vi "MotorTypeParametersMaxMin.vi"(11 "MotorType":T2) -> (2 "Min":T1, 3 "Max":T1)   [LabVIEW 2019, in "CubeMarsBLDClib.lvlib"]
uses:
  CubeMarsBLDClib.lvlib
  MotorType.ctl
  MotorParameters.ctl
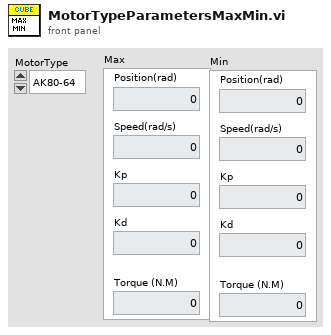
[diagram p1: front panel]
types:
  T1 = typedef "CubeMarsBLDClib.lvlib/MotorParameters.ctl" = cluster{"Position(rad)":dbl, "Speed(rad/s)":dbl, "Kp":dbl, "Kd":dbl, "Torque (N.M)":dbl}
  T2 = typedef "CubeMarsBLDClib.lvlib/MotorType.ctl" = enum16{"AK80-64", "AK80-9", "AK80-8", "AK80-6", "AK70-10", "AK60-6", "AK10-9"}
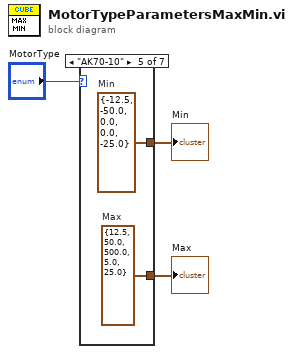
[diagram p0: block diagram]
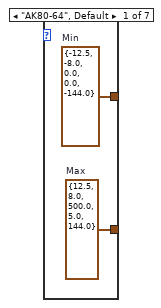
[diagram p2: hidden frame]
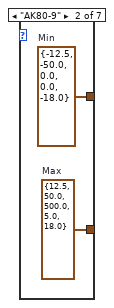
[diagram p3: hidden frame]
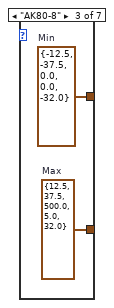
[diagram p4: hidden frame]
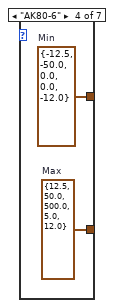
[diagram p5: hidden frame]
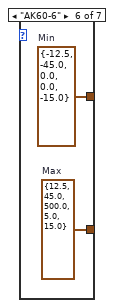
[diagram p6: hidden frame]
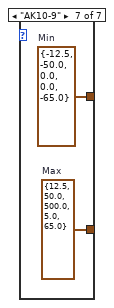
[diagram p7: hidden frame]
diagram:
  n1 = case shown="\"AK70-10\"" "MotorType" {
    tunnel: [w5 w7 w9 w11 w12 w15 w17] -> w1
    tunnel: [w4 w6 w8 w10 w13 w14 w16] -> w2
    frame "AK80-64", Default {
      w4 = T1 {"Position(rad)"=12.5, "Speed(rad/s)"=8.0, "Kp"=500.0, "Kd"=5.0, "Torque (N.M)"=144.0}  # Max
      w5 = T1 {"Position(rad)"=-12.5, "Speed(rad/s)"=-8.0, "Kp"=0.0, "Kd"=0.0, "Torque (N.M)"=-144.0}  # Min
    }
    frame "AK80-9" {
      w6 = T1 {"Position(rad)"=12.5, "Speed(rad/s)"=50.0, "Kp"=500.0, "Kd"=5.0, "Torque (N.M)"=18.0}  # Max
      w7 = T1 {"Position(rad)"=-12.5, "Speed(rad/s)"=-50.0, "Kp"=0.0, "Kd"=0.0, "Torque (N.M)"=-18.0}  # Min
    }
    frame "AK80-8" {
      w8 = T1 {"Position(rad)"=12.5, "Speed(rad/s)"=37.5, "Kp"=500.0, "Kd"=5.0, "Torque (N.M)"=32.0}  # Max
      w9 = T1 {"Position(rad)"=-12.5, "Speed(rad/s)"=-37.5, "Kp"=0.0, "Kd"=0.0, "Torque (N.M)"=-32.0}  # Min
    }
    frame "AK80-6" {
      w10 = T1 {"Position(rad)"=12.5, "Speed(rad/s)"=50.0, "Kp"=500.0, "Kd"=5.0, "Torque (N.M)"=12.0}  # Max
      w11 = T1 {"Position(rad)"=-12.5, "Speed(rad/s)"=-50.0, "Kp"=0.0, "Kd"=0.0, "Torque (N.M)"=-12.0}  # Min
    }
    frame "AK70-10" {
      w13 = T1 {"Position(rad)"=12.5, "Speed(rad/s)"=50.0, "Kp"=500.0, "Kd"=5.0, "Torque (N.M)"=25.0}  # Max
      w12 = T1 {"Position(rad)"=-12.5, "Speed(rad/s)"=-50.0, "Kp"=0.0, "Kd"=0.0, "Torque (N.M)"=-25.0}  # Min
    }
    frame "AK60-6" {
      w14 = T1 {"Position(rad)"=12.5, "Speed(rad/s)"=45.0, "Kp"=500.0, "Kd"=5.0, "Torque (N.M)"=15.0}  # Max
      w15 = T1 {"Position(rad)"=-12.5, "Speed(rad/s)"=-45.0, "Kp"=0.0, "Kd"=0.0, "Torque (N.M)"=-15.0}  # Min
    }
    frame "AK10-9" {
      w16 = T1 {"Position(rad)"=12.5, "Speed(rad/s)"=50.0, "Kp"=500.0, "Kd"=5.0, "Torque (N.M)"=65.0}  # Max
      w17 = T1 {"Position(rad)"=-12.5, "Speed(rad/s)"=-50.0, "Kp"=0.0, "Kd"=0.0, "Torque (N.M)"=-65.0}  # Min
    }
  }
  "Max" <- w2
  "Min" <- w1
